vi "Calculate_Angles_for_Subtrack_Displ-1.vi"(5 "[IN] Index of subtrack":i32, 6 "[IN] Subtrack":dbl[](array[numeric]), 7 "[IN] Index of \"11\" Dis-\nplacement in Subtrack":i32, 8 "[IN] Reverse Displ or Not":bool[](array[boolean]), 9 "[IN] Array with Angles \nBetween Displacement":dbl[](array[numeric])) -> (2 "[OUT] Reverse displacement or not":bool[](array[boolean]), 3 "[OUT] Angles betwe\nen two displacements":dbl[](array[numeric]))   [LabVIEW 2013]
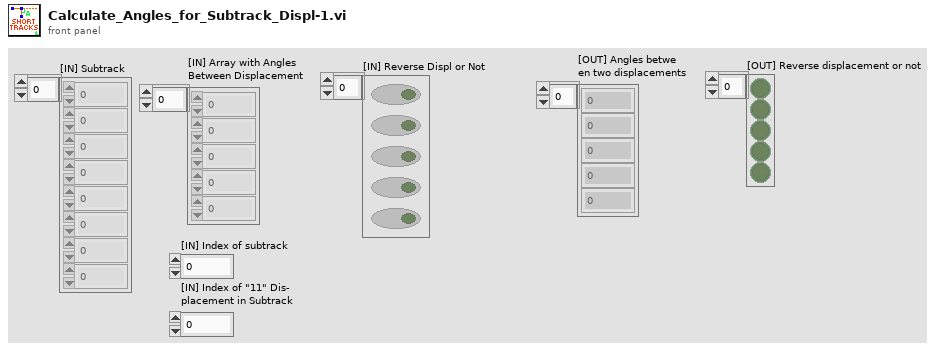
[diagram p1: front panel]
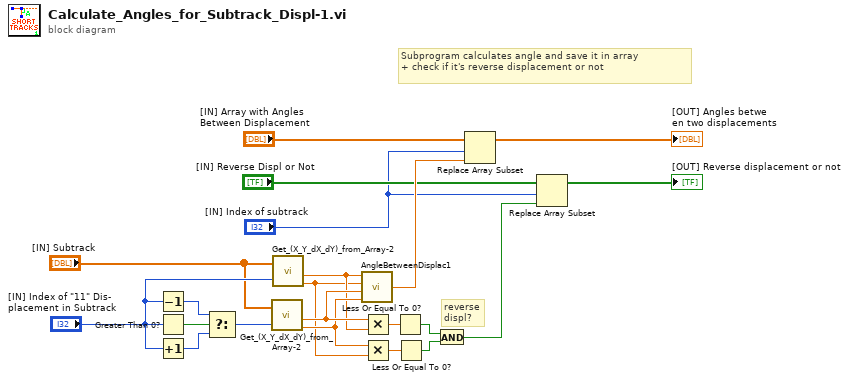
[diagram p0: block diagram]
diagram:
  # "Subprogram calculates angle and save it in array \n+ check if it's reverse displacement or not"
  # "reverse \ndispl?"
  n1 = Decrement(x="[IN] Index of \"11\" Dis-\nplacement in Subtrack") -> (x-1=w20:i32)
  n2 = Greater Than 0?(x="[IN] Index of \"11\" Dis-\nplacement in Subtrack") -> (x > 0?=w21:bool)
  n3 = Increment(x="[IN] Index of \"11\" Dis-\nplacement in Subtrack") -> (x+1=w19:i32)
  n4 = Select(t=w20, s=w21, f=w19) -> (s? t:f=w16:i32)
  n5 = call "Get_(X_Y_dX_dY)_from_Array-2.vi"("(X,Y,dX,dY)"="[IN] Subtrack", "Index of Displacement"=w16) -> ("dX"=w11:dbl, "dY"=w10:dbl)  [unwired: 2 out]
  n6 = call "Get_(X_Y_dX_dY)_from_Array-2.vi"("(X,Y,dX,dY)"="[IN] Subtrack", "Index of Displacement"="[IN] Index of \"11\" Dis-\nplacement in Subtrack") -> ("dX"=w9:dbl, "dY"=w8:dbl)  [unwired: 2 out]
  n7 = call "AngleBetweenDisplac1.vi"("dY 2"=w10, "dX 2"=w11, "dY 1"=w8, "dX 1"=w9) -> ("angle in degrees"=w6:dbl)
  n8 = Multiply(x=w11, y=w9) -> (x*y=w15:dbl)
  n9 = Multiply(x=w10, y=w8) -> (x*y=w14:dbl)
  n10 = Less Or Equal To 0?(x=w15) -> (x <= 0?=w12:bool)
  n11 = Less Or Equal To 0?(x=w14) -> (x <= 0?=w13:bool)
  n12 = And(x=w12, y=w13) -> (x .and. y?=w3:bool)
  n13 = Replace Array Subset(array="[IN] Array with Angles \nBetween Displacement", new element=w6, index="[IN] Index of subtrack") -> (→"[OUT] Angles betwe\nen two displacements":dbl[])
  n14 = Replace Array Subset(array="[IN] Reverse Displ or Not", new element=w3, index="[IN] Index of subtrack") -> (→"[OUT] Reverse displacement or not":bool[])
